vi "S3.vi"(1 "Input array":bool[](array[boolean])) -> (0 "Array":bool[](array[boolean]))   [LabVIEW 2013]
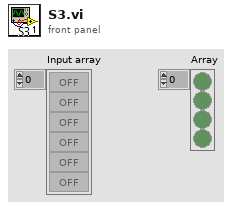
[diagram p1: front panel]
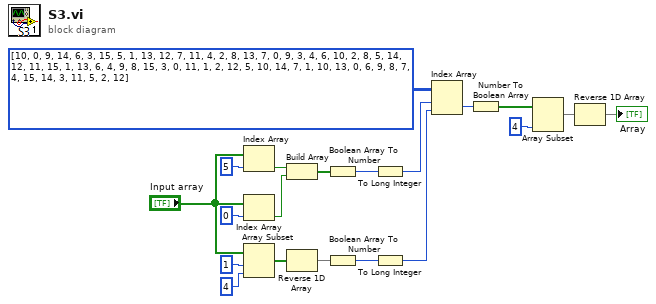
[diagram p0: block diagram]
diagram:
  n1 = Index Array(array="Input array", index=5) -> (element=w3:bool)
  n2 = Index Array(array="Input array", index=0) -> (element=w2:bool)
  n3 = Array Subset(array="Input array", index=1, length=4) -> (w11:bool[])
  n4 = Build Array(w3, w2) -> (w1:bool[])
  n5 = Reverse 1D Array(array=w11) -> (reversed array=w10:bool[])
  n6 = Boolean Array To Number(Boolean array=w1) -> (number=w15:u32)
  n7 = Boolean Array To Number(Boolean array=w10) -> (number=w14:u32)
  n8 = To Long Integer(number=w15) -> (32bit integer=w9:i32)
  n9 = To Long Integer(number=w14) -> (32bit integer=w8:i32)
  n10 = Index Array(array=u8[][] [[10, 0, 9, 14, 6, 3, 15, 5, 1, 13, 12, 7, 11, 4, 2, 8], [13, 7, 0, 9, 3, 4, 6, 10, 2, 8, 5, 14, 12, 11, 15, 1], [13, 6, 4, 9, 8, 15, 3, 0, 11, 1, 2, 12, 5, 10, 14, 7], [1, 10, 13, 0, 6, 9, 8, 7, 4, 15, 14, 3, 11, 5, 2, 12]], index (row)=w9, index (col)=w8) -> (element=w20:u8)
  n11 = Number To Boolean Array(number=w20) -> (Boolean array=w19:bool[])
  n12 = Array Subset(array=w19, length=4) -> (w7:bool[])  [unwired: 1 in]
  n13 = Reverse 1D Array(array=w7) -> (reversed array=→"Array":bool[])
